vi "Configure Session.vi"(8 "error in":errorcluster, 11 "Plugin in":refnum<class "Sift TDMS Uploader.lvclass">) -> (0 "error out":errorcluster, 3 "Plugin out":refnum<class "Sift TDMS Uploader.lvclass">)   [LabVIEW 2024, in "Sift TDMS Uploader.lvlib" / "Sift TDMS Uploader.lvclass"]
uses:
  Sift TDMS Uploader.lvclass
  C:/Program Files/National Instruments/LabVIEW 2024/vi.lib/FlexLogger/SDK/PluginSDK.lvlibp/PEFClasses/SDK/Plugin/Plugin.lvclass
  Sift TDMS Uploader.lvclass/Sift TDMS Uploader.ctl
  <vilib>/FlexLogger/SDK/PluginSDK.lvlibp/PEFClasses/SDK/Plugin/ParameterAccess/Read String.vi
  <vilib>/FlexLogger/SDK/PluginSDK.lvlibp/PEFClasses/SDK/Plugin/Plugin.lvclass
  C:/Program Files/National Instruments/LabVIEW 2024/vi.lib/FlexLogger/SDK/PluginSDK.lvlibp/PEFClasses/SDK/Processing Element/Processing Element.lvclass
  C:/Users/Alex luCK/Documents/Projects/sift-labview/plugins/flexlogger/Sift TDMS Uploader/Sift TDMS Uploader.lvclass
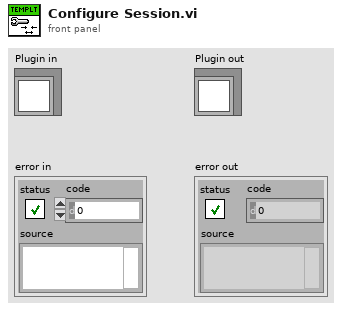
[diagram p1: front panel]
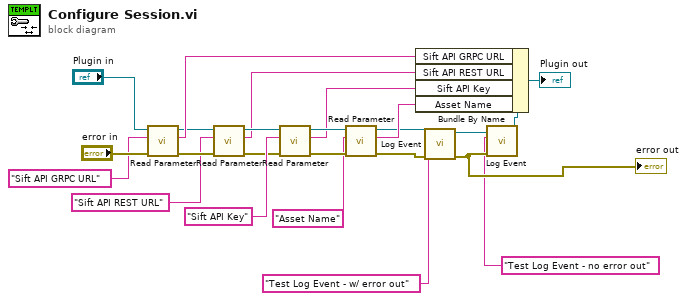
[diagram p0: block diagram]
diagram:
  n1 = call-poly <vilib>:"Read Parameter.vi"("error in (no error)"="error in", "Name"="Sift API GRPC URL", "Plugin in"="Plugin in") -> ("error out"=w11:errorcluster, "Value"=w18:string, "Plugin out"=w12:refnum<class "Sift TDMS Uploader.lvclass">)  [unwired: 5 in, 1 out]
  n2 = call-poly <vilib>:"Read Parameter.vi"("error in (no error)"=w11, "Name"="Sift API REST URL", "Plugin in"=w12) -> ("error out"=w13:errorcluster, "Value"=w8:string, "Plugin out"=w14:refnum<class "Sift TDMS Uploader.lvclass">)  [unwired: 5 in, 1 out]
  n3 = call-poly <vilib>:"Read Parameter.vi"("error in (no error)"=w13, "Name"="Sift API Key", "Plugin in"=w14) -> ("error out"=w24:errorcluster, "Value"=w9:string, "Plugin out"=w23:refnum<class "Sift TDMS Uploader.lvclass">)  [unwired: 5 in, 1 out]
  n4 = call-poly <vilib>:"Read Parameter.vi"("error in (no error)"=w24, "Name"="Asset Name", "Plugin in"=w23) -> ("error out"=w7:errorcluster, "Value"=w19:string, "Plugin out"=w6:refnum<class "Sift TDMS Uploader.lvclass">)  [unwired: 5 in, 1 out]
  n5 = call <vilib>:"Log Event.vi"("error in (no error)"=w7, "Message"="Test Log Event - w/ error out", "Plugin in"=w6) -> ("error out"=w3:errorcluster, "Plugin out"=w5:refnum<class "Sift TDMS Uploader.lvclass">)  [unwired: 7 in]
  "error out" <- w3
  n6 = call <vilib>:"Log Event.vi"("error in (no error)"=w3, "Message"="Test Log Event - no error out", "Plugin in"=w5) -> ("Plugin out"=w4:refnum<class "Sift TDMS Uploader.lvclass">)  [unwired: 7 in, 1 out]
  n7 = Bundle By Name(cluster=w4, "Sift API GRPC URL"=w18, "Sift API REST URL"=w8, "Sift API Key"=w9, "Asset Name"=w19) -> (→"Plugin out":refnum<class "Sift TDMS Uploader.lvclass">)
